vi "IECMemory.constructor.vi"(0 "name":string, 2 "data in":string, 5 "error in(no error)":errorcluster) -> (14 "i ref out":refnum<vi>, 16 "data out":string, 19 "error out":errorcluster)   [LabVIEW 2014, in "IECMemory.lvlib"]
doc: "class encapsulates the driver for the Mainz E-Lab memory (pattern generator)\n\nauthor: Frank Herfurth, CERN\n\nLicense Agreement for this software:\n\nCopyright (C)\nGesellschaft für Schwerionenforschung, GSI\nPlanckstr. 1\n64291 Darmstadt\nGermany\n\nContact: D.Beck@gsi.de \n\nThis program is free software; you can redistribute it and/or modify it under the terms of the \nGNU General Public License as published by the Free Software Foundation; either version 2 of \nthe license, or (at your option) any later version.\n\nThis program is distributed in the hope that it will be useful, but WITHOUT ANY WARRANTY; \nwithout even the implied warranty of MERCHANTABILITY or FITNESS FOR A PARTICULAR PURPOSE. See the GNU General License for more details (http://www.gnu.org).\n\nGesellschaft für Schwerionenforschung, GSI\nPlanckstr. 1, 64291 Darmstadt, Germany\nFor all questions and ideas contact: M.Richter@gsi.de, H.Brand@gsi.de or D.Beck@gsi.de.\nLast update: 16-JUN-2004"
uses:
  IECMemory.lvlib
  CSCore/BaseProcess/BaseProcess.lvlib
  CSCore/CSSystem/CSSystemLib/CSSystemLib.lvlib
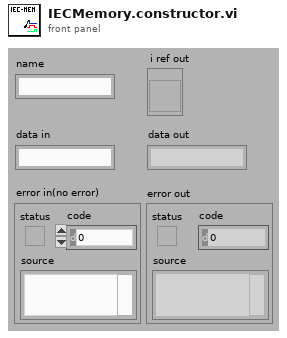
[diagram p1: front panel]
types:
  T1 = enum16{"SetAttribute", "GetAttribute", "CreateAttribute", "DestroyAttribute", "DestroyAllAtributes"}
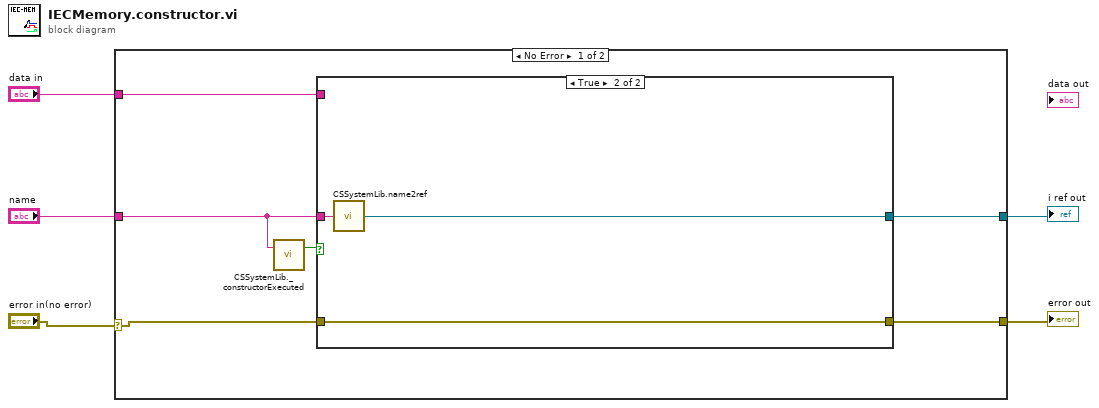
[diagram p0: block diagram]
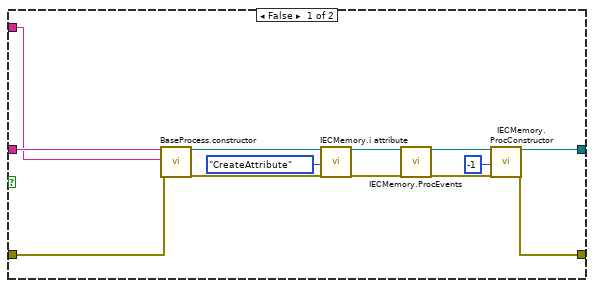
[diagram p2: hidden frame]
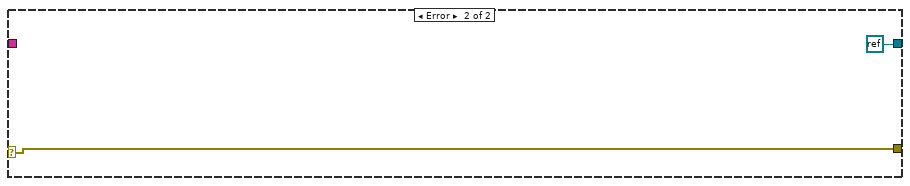
[diagram p3: hidden frame]
diagram:
  n1 = case shown="No Error" "error in(no error)" {
    selector: "error in(no error)" -> [w11 w29]
    tunnel: "name" -> [w8 _]
    tunnel: "data in" -> [w10 _]
    tunnel: [w7 w29] -> w2
    tunnel: [w6 refnum<k0> refnum] -> w1
    frame No Error {
      n2 = call "CSSystemLib._constructorExecuted.vi"("name"=w8) -> ("constructor executed?"=w9:bool)  [unwired: 18 in]
      n3 = case shown="True" w9 {
        tunnel: w11 -> [w24 w27]
        tunnel: w8 -> [w20 w26]
        tunnel: [w15 w25] -> w6
        tunnel: [w14 w27] -> w7
        tunnel: w10 -> [w12 _]
        frame False {
          n4 = call "BaseProcess.constructor.vi"("name"=w20, "data in"=w12, "error in (no error)"=w24) -> ("i ref out"=w23:refnum<vi>, "error out"=w22:errorcluster)  [unwired: 14 in, 1 out]
          n5 = call "IECMemory.i attribute.vi"("VI Refnum"=w23, "Action"=T1."CreateAttribute", "error in (no error)"=w22) -> ("VI Refnum out"=w19:refnum<vi>, "error out"=w18:errorcluster)  [unwired: 14 in, 1 out]
          n6 = call "IECMemory.ProcEvents.vi"("i ref in"=w19, "error in"=w18) -> ("i ref out"=w17:refnum<vi>, "error out"=w16:errorcluster)  [unwired: 16 in]
          n7 = call "IECMemory.ProcConstructor.vi"("i ref in"=w17, "ms timeout (100)"=-1, "error in (no error)"=w16) -> ("i ref out"=w15:refnum<vi>, "error out"=w14:errorcluster)  [unwired: 14 in, 1 out]
        }
        frame True {
          n8 = call "CSSystemLib.name2ref.vi"("name"=w26) -> ("obj refnum"=w25:refnum<vi>)
        }
      }
    }
    frame Error {
    }
  }
  "i ref out" <- w1
  "error out" <- w2
